vi "User_Name.vi"() -> (0 "User Name":string)   [LabVIEW 2020]
uses:
  Anemometry/Anemometry Sub Vis/Globals/Trav_pos_global.vi
  Anemometry/Anemometry Sub Vis/Globals/Preference_global.vi
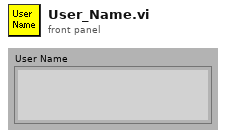
[diagram p1: front panel]
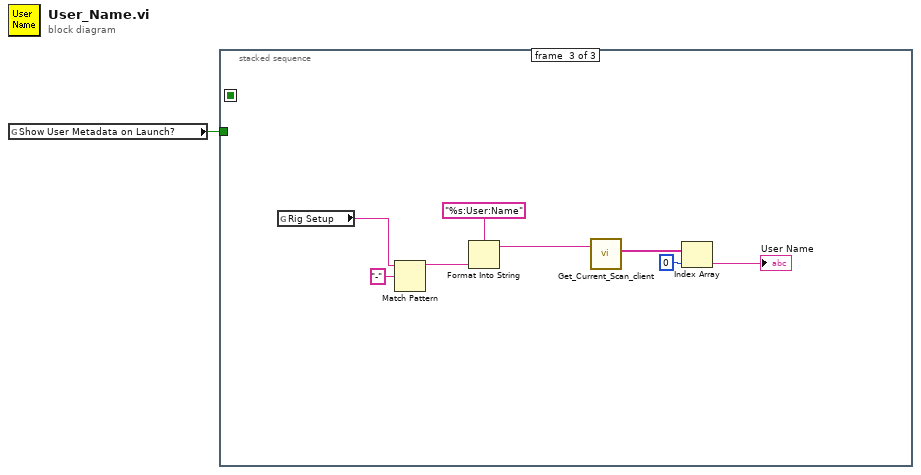
[diagram p0: block diagram]
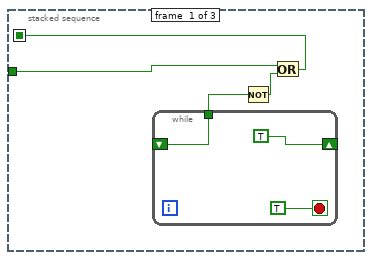
[diagram p2: hidden frame]
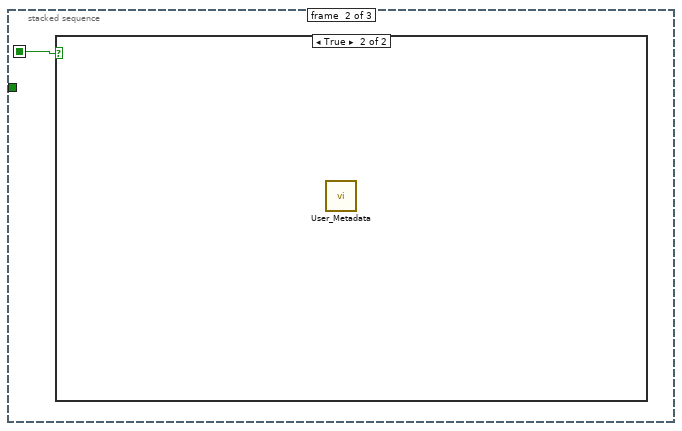
[diagram p3: hidden frame]
diagram:
  n1 = global read "Trav_pos_global.vi" "Show User Metadata on Launch?"() -> (w1:bool)
  n2 = stacked-sequence {
    seq-local: [w4 _ _] -> [_ w9 _]
    tunnel: w1 -> [w2 _ _]
    frame #0 {
      n3 = while {
        shift-right: [TRUE] -> _
        shift-left: _ -> [w6]
        tunnel: [w6] -> w5
        stop <- TRUE stop-if-true
      }
      n4 = Not(x=w5) -> (.not. x?=w3:bool)
      n5 = Or(x=w2, y=w3) -> (x .or. y?=w4:bool)
    }
    frame #1 {
      n6 = case shown="True" w9 {
        frame False {
        }
        frame True {
          n7 = call "User_Metadata.vi"() -> ()  [unwired: 9 out]
        }
      }
    }
    frame #2 {
      n8 = global read "Preference_global.vi" "Rig Setup"() -> (w12:string)
      n9 = Match Pattern(string=w12, regular expression="-") -> (before substring=w11:string)  [unwired: 4 out]
      n10 = Format Into String(format string="%s:User:Name" ("Format String"), w11) -> (resulting string=w10:string)  [unwired: 2 in, 1 out]
      n11 = call "Get_Current_Scan_client.vi"("singleChannel"=w10) -> ("String values"=w16:string[])  [unwired: 2 in, 2 out]
      n12 = Index Array(array=w16, index=0) -> (element=→"User Name":string)
    }
  }
